vi "Library Path_LLLB2.vi"(11 "File Path":path) -> (2 "Is in llb?":bool, 3 "llb path":path)   [LabVIEW 2023]
doc: "Determine if VI is in llb and return llb path. Path out is empty if not llb."
uses:
  <userlib>/_OpenG.lib/file/file.llb/openg_file.lvlib
  <userlib>/_OpenG.lib/file/file.llb/Strip Path Extension - String__ogtk.vi
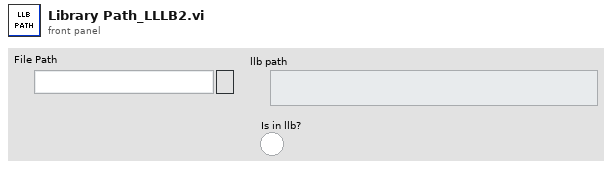
[diagram p1: front panel]
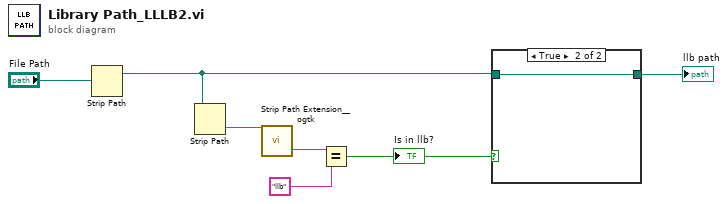
[diagram p0: block diagram]
diagram:
  n1 = Strip Path(path="File Path") -> (stripped path=w1:path)  [unwired: 1 out]
  n2 = Strip Path(path=w1) -> (name=w7:string)  [unwired: 1 out]
  n3 = call-poly <userlib>:"Strip Path Extension__ogtk.vi"("path"=w7) -> ("extension"=w6:string)  [unwired: 1 out]
  n4 = Equal?(x=w6, y="llb") -> (x = y?=w2:bool)
  "Is in llb?" <- w2
  n5 = case shown="True" w2 {
    tunnel: [_ w8] -> w4
    tunnel: w1 -> [_ w8]
    frame False {
    }
    frame True {
    }
  }
  "llb path" <- w4
